vi "SetCalibrationData.vi"(0 "AIs in":refnum<class "AI.lvclass">[](array[class]), 5 "data":T1) -> (4 "AIs out":refnum<class "AI.lvclass">[](array[class]))   [LabVIEW 2019, in "Stand.lvclass"]
uses:
  Stand.lvclass
  TypeDef/CalibrationData.ctl
  TypeDef/GUI Setting Channel.ctl
  TypeDef/GUI AI Ranges.ctl
  TypeDef/Scale Data.ctl
  AI_class/AI.lvclass
  PiecedLinearScale_class/Scale_PiecedLinear.lvclass
  TypeDef/ConfigAnalogComp.ctl
  AI_class/AI Alarm Type.ctl
  PiecedLinearScale_class/Scale_PiecedLinear.lvclass/Scale_PiecedLinear.ctl
  AI_class/AI.lvclass/AI.ctl
  AnalogComparator_class/AnalogComparator.lvclass/AnalogComparator.ctl
  AnalogComparator_class/SetConfig.vi
  AnalogComparator_class/AnalogComparator.lvclass
panel:
  # "SCALED"
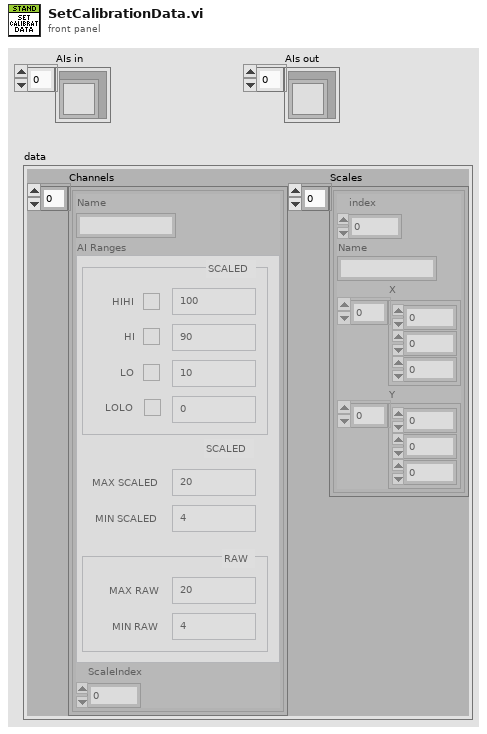
[diagram p1: front panel]
types:
  T1 = typedef "CalibrationData.ctl" = cluster{"Channels":T2[], "Scales":T4[]}
  T2 = typedef "GUI Setting Channel.ctl" = cluster{"Name":string, "AI Ranges":T3, "ScaleIndex":u32}
  T3 = typedef "GUI AI Ranges.ctl" = cluster{"HI":bool, "HIHI":bool, "LO":bool, "LOLO":bool, "HIHI VAL":dbl, "HI VAL":dbl, "LO VAL":dbl, "LOLO VAL":dbl, "MAX RAW":dbl, "MIN RAW":dbl, "MAX SCALED":dbl, "MIN SCALED":dbl}
  T4 = typedef "Scale Data.ctl" = cluster{"index":i32, "Name":string, "X":dbl[], "Y":dbl[]}
  T5 = typedef "AnalogComparator.lvclass/AI Alarm Type.ctl" = enum16{"RAW MAX", "RAW MIN", "HIHI", "HI", "LO", "LOLO"}
  T6 = typedef "ConfigAnalogComp.ctl" = cluster{"Threshold":dbl, "Hysteresis":dbl, "Invert":bool, "Enable":bool, "LockEn":bool}
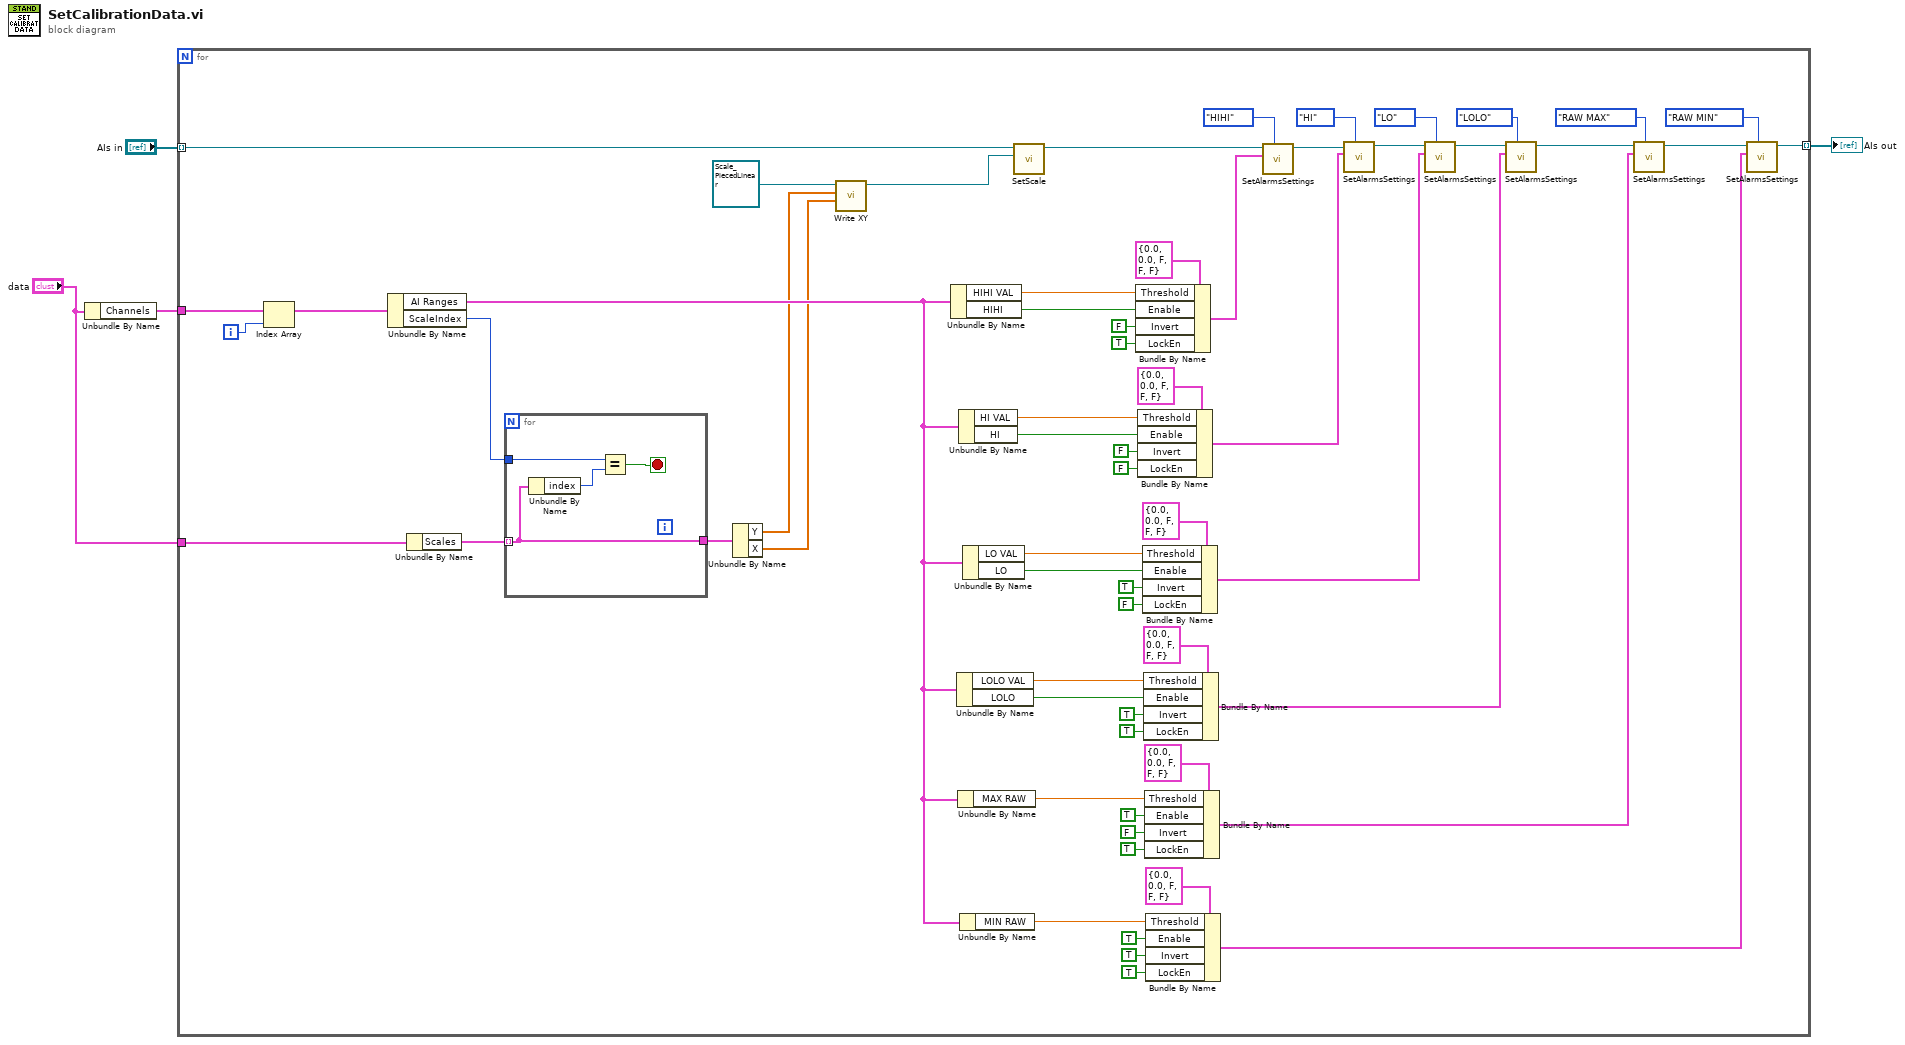
[diagram p0: block diagram]
diagram:
  n1 = Unbundle By Name("data") -> ("Channels"=w2:T2[])
  n2 = for {
    tunnel: "AIs in" -> [w66] mode=indexing
    tunnel: [w24] -> w3 mode=indexing
    tunnel: w2 -> [w63]
    tunnel: "data" -> [w11]
    i -> [w5]
    n3 = Index Array(array=w63, index=w5) -> (element=w6:T2)
    n4 = Unbundle By Name(w6) -> ("AI Ranges"=w32:T3, "ScaleIndex"=w10:u32)
    n5 = Unbundle By Name(w11) -> ("Scales"=w12:T4[])
    n6 = for {
      tunnel: w12 -> [w67] mode=indexing
      tunnel: w10 -> [w70]
      tunnel: [w67] -> w9
      stop <- w68 stop-if-true
      n7 = Unbundle By Name(w67) -> ("index"=w69:i32)
      n8 = Equal?(x=w70, y=w69) -> (x = y?=w68:bool)
    }
    n9 = Unbundle By Name(w9) -> ("Y"=w8:dbl[], "X"=w7:dbl[])
    n10 = call "Write XY.vi"("X"=w7, "Y"=w8, "Scale_PiecedLinear in"=refnum<class "Scale_PiecedLinear.lvclass"> refnum) -> ("Scale_PiecedLinear out"=w64:refnum<class "Scale_PiecedLinear.lvclass">)  [unwired: 8 in]
    n11 = Unbundle By Name(w32) -> ("HIHI VAL"=w61:dbl, "HIHI"=w60:bool)
    n12 = Unbundle By Name(w32) -> ("LOLO VAL"=w44:dbl, "LOLO"=w45:bool)
    n13 = Unbundle By Name(w32) -> ("MAX RAW"=w41:dbl)
    n14 = Unbundle By Name(w32) -> ("HI VAL"=w54:dbl, "HI"=w55:bool)
    n15 = Unbundle By Name(w32) -> ("MIN RAW"=w34:dbl)
    n16 = Unbundle By Name(w32) -> ("LO VAL"=w51:dbl, "LO"=w50:bool)
    n17 = call "SetScale.vi"("Scale"=w64, "Sig_AI in"=w66) -> ("Sig_AI out"=w31:refnum<class "AI.lvclass">)  [unwired: 9 in]
    n18 = Bundle By Name(cluster=T6 {"Threshold"=0.0, "Hysteresis"=0.0, "Invert"=FALSE, "Enable"=FALSE, "LockEn"=FALSE} ("SettinganalogComp"), "Threshold"=w61, "Enable"=w60, "Invert"=FALSE, "LockEn"=TRUE) -> (w30:T6)
    n19 = Bundle By Name(cluster=T6 {"Threshold"=0.0, "Hysteresis"=0.0, "Invert"=FALSE, "Enable"=FALSE, "LockEn"=FALSE} ("SettinganalogComp"), "Threshold"=w54, "Enable"=w55, "Invert"=FALSE, "LockEn"=FALSE) -> (w23:T6)
    n20 = Bundle By Name(cluster=T6 {"Threshold"=0.0, "Hysteresis"=0.0, "Invert"=FALSE, "Enable"=FALSE, "LockEn"=FALSE} ("SettinganalogComp"), "Threshold"=w51, "Enable"=w50, "Invert"=TRUE, "LockEn"=FALSE) -> (w22:T6)
    n21 = Bundle By Name(cluster=T6 {"Threshold"=0.0, "Hysteresis"=0.0, "Invert"=FALSE, "Enable"=FALSE, "LockEn"=FALSE} ("SettinganalogComp"), "Threshold"=w44, "Enable"=w45, "Invert"=TRUE, "LockEn"=TRUE) -> (w21:T6)
    n22 = Bundle By Name(cluster=T6 {"Threshold"=0.0, "Hysteresis"=0.0, "Invert"=FALSE, "Enable"=FALSE, "LockEn"=FALSE} ("SettinganalogComp"), "Threshold"=w41, "Enable"=TRUE, "Invert"=FALSE, "LockEn"=TRUE) -> (w20:T6)
    n23 = Bundle By Name(cluster=T6 {"Threshold"=0.0, "Hysteresis"=0.0, "Invert"=FALSE, "Enable"=FALSE, "LockEn"=FALSE} ("SettinganalogComp"), "Threshold"=w34, "Enable"=TRUE, "Invert"=TRUE, "LockEn"=TRUE) -> (w19:T6)
    n24 = call "SetAlarmsSettings.vi"("TYPE"=AI_Alarm_Type."HIHI", "SettinganalogComp"=w30, "Sig_AI in"=w31) -> ("Sig_AI out"=w29:refnum<class "AI.lvclass">)  [unwired: 8 in]
    n25 = call "SetAlarmsSettings.vi"("TYPE"=AI_Alarm_Type."HI", "SettinganalogComp"=w23, "Sig_AI in"=w29) -> ("Sig_AI out"=w28:refnum<class "AI.lvclass">)  [unwired: 8 in]
    n26 = call "SetAlarmsSettings.vi"("TYPE"=AI_Alarm_Type."LO", "SettinganalogComp"=w22, "Sig_AI in"=w28) -> ("Sig_AI out"=w27:refnum<class "AI.lvclass">)  [unwired: 8 in]
    n27 = call "SetAlarmsSettings.vi"("TYPE"=AI_Alarm_Type."LOLO", "SettinganalogComp"=w21, "Sig_AI in"=w27) -> ("Sig_AI out"=w26:refnum<class "AI.lvclass">)  [unwired: 8 in]
    n28 = call "SetAlarmsSettings.vi"("TYPE"=AI_Alarm_Type."RAW MAX", "SettinganalogComp"=w20, "Sig_AI in"=w26) -> ("Sig_AI out"=w25:refnum<class "AI.lvclass">)  [unwired: 8 in]
    n29 = call "SetAlarmsSettings.vi"("TYPE"=AI_Alarm_Type."RAW MIN", "SettinganalogComp"=w19, "Sig_AI in"=w25) -> ("Sig_AI out"=w24:refnum<class "AI.lvclass">)  [unwired: 8 in]
  }
  "AIs out" <- w3
